vi "Open DSFConfig Data.vi"(8 "error in (no error)":errorcluster, 10 "create file if necessary (T)":bool=TRUE, 11 "configuration file path":path) -> (0 "error out":errorcluster, 2 "file created?":bool, 3 "refnum":T2, 4 "version":T1)   [LabVIEW 2017, in "DSF Configuration API.lvlib"]
doc: "Opens a reference to the configuration data found in a platform-independent configuration file."
uses:
  DSF Configuration API.lvlib
  Controls/DSF Config Data RefNum.ctl
  Controls/Version Info.ctl
  Private/Controls/Session/Config Data.ctl
  Private/Controls/DSF File Format/DSF Config.ctl
  Private/Controls/DSF File Format/DSF Plugin.ctl
  Controls/DSF Plugin Info.ctl
  Controls/DSF Timing Info.ctl
  Private/Controls/DSF File Format/DSF Group.ctl
  Controls/DSF Group Info.ctl
  Private/Controls/DSF File Format/DSF Transfer.ctl
  Controls/DSF Transfer Info.ctl
  Private/Controls/DSF File Format/DSF Channel.ctl
  Controls/DSF Channel Info.ctl
  Private/Controls/DSF File Format/DSF Settings.ctl
  Controls/DSF Settings Info.ctl
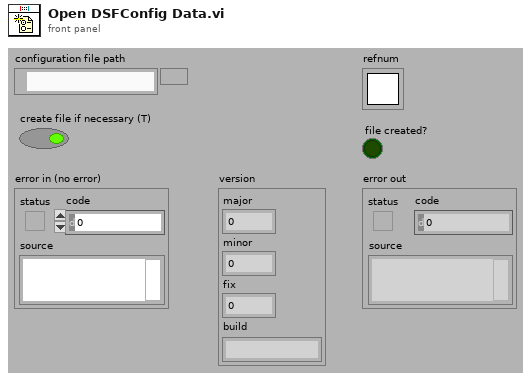
[diagram p1: front panel]
types:
  T1 = typedef "DSF Configuration API.lvlib/Version Info.ctl" = cluster{"major":u32, "minor":u32, "fix":u32, "build":string}
  T2 = typedef "DSF Configuration API.lvlib/DSF Config Data RefNum.ctl" = refnum<k1>
  T3 = typedef "DSF Configuration API.lvlib/Config Data.ctl" = cluster{"dsf configuration":T4, "path":path, "dirty":bool}
  T4 = typedef "DSF Configuration API.lvlib/DSF Config.ctl" = cluster{"dsfversion":T1, "version":T1, "plugins":T5[], "groups":T8[], "transfers":T10[], "channels":T12[], "settings":T14[]}
  T5 = typedef "DSF Configuration API.lvlib/DSF Plugin.ctl" = cluster{"id":string, "values":T6}
  T6 = typedef "DSF Configuration API.lvlib/DSF Plugin Info.ctl" = cluster{"type":string, "timing":T7, "group ids":string[], "settings id":string}
  T7 = typedef "DSF Configuration API.lvlib/DSF Timing Info.ctl" = cluster{"decimation":i32, "offset":i32}
  T8 = typedef "DSF Configuration API.lvlib/DSF Group.ctl" = cluster{"id":string, "values":T9}
  T9 = typedef "DSF Configuration API.lvlib/DSF Group Info.ctl" = cluster{"direction":i32, "timing":T7, "transfer ids":string[], "settings id":string}
  T10 = typedef "DSF Configuration API.lvlib/DSF Transfer.ctl" = cluster{"id":string, "values":T11}
  T11 = typedef "DSF Configuration API.lvlib/DSF Transfer Info.ctl" = cluster{"byte order":i32, "channel ids":string[], "settings id":string}
  T12 = typedef "DSF Configuration API.lvlib/DSF Channel.ctl" = cluster{"id":string, "values":T13}
  T13 = typedef "DSF Configuration API.lvlib/DSF Channel Info.ctl" = cluster{"count":i32, "offset":i32, "data type":i32, "resource path":string, "settings id":string}
  T14 = typedef "DSF Configuration API.lvlib/DSF Settings.ctl" = cluster{"id":string, "values":T15}
  T15 = typedef "DSF Configuration API.lvlib/DSF Settings Info.ctl" = cluster{"key":string, "value":string}[]
  T16 = typedef "DSF Configuration API.lvlib/Config Queue.ctl" = refnum<queue>
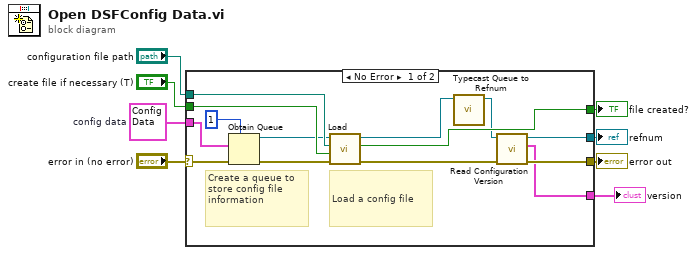
[diagram p0: block diagram]
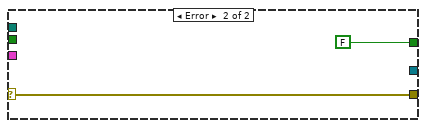
[diagram p2: hidden frame]
diagram:
  w2 = T3 {"dsf configuration"={"dsfversion"={"major"=0, "minor"=0, "fix"=0, "build"=""}, "version"={"major"=0, "minor"=0, "fix"=0, "build"=""}, "plugins"=[], "groups"=[], "transfers"=[], "channels"=[], "settings"=[]}, "path"=path "", "dirty"=FALSE}  # config data
  n1 = case shown="No Error" "error in (no error)" {
    selector: "error in (no error)" -> [w17 w24]
    tunnel: "configuration file path" -> [w22 _]
    tunnel: "create file if necessary (T)" -> [w21 _]
    tunnel: [w19 FALSE ("file created?")] -> w4
    tunnel: [w12 w24] -> w5
    tunnel: w2 -> [w16 _]
    tunnel: [w10 _] -> w3
    tunnel: [w9 _] -> w1
    frame No Error {
      # "Load a config file"
      # "Create a queue to store config file information"
      n2 = Obtain Queue(max queue size (-1, unlimited)=1, element data type=w16, error in (no error)=w17) -> (queue out=w13:refnum<queue>, error out=w15:errorcluster)  [unwired: 2 in, 1 out]
      n3 = call "Load.vi"("error in (no error)"=w15, "create file if necessary? (T)"=w21, "configuration file path"=w22, "queue in"=w13) -> ("error out"=w20:errorcluster, "file created?"=w19:bool, "queue out"=w14:T16)  [unwired: 5 out]
      n4 = call "Typecast Queue to Refnum.vi"("queue in"=w14) -> ("refnum out"=w11:T2)  [unwired: 10 in]
      n5 = call "Read Configuration Version.vi"("error in (no error)"=w20, "refnum"=w11) -> ("error out"=w12:errorcluster, "version"=w9:T1, "refnum out"=w10:T2)  [unwired: 7 in]
    }
    frame Error {
    }
  }
  "error out" <- w5
  "file created?" <- w4
  "refnum" <- w3
  "version" <- w1
